vi "read.vi"(8 "error in (no error)":errorcluster caption="错误输入（无错误）", 11 "TCP_client 输入":refnum<class "TCP_client.lvclass">) -> (0 "error out":errorcluster caption="错误输出", 2 "read":string, 3 "TCP_client 输出":refnum<class "TCP_client.lvclass">)   [LabVIEW 2022 SP3, in "update.lvlib" / "TCP_client.lvclass"]
uses:
  TCP_client.lvclass
  TCP_client.lvclass/TCP_client.ctl
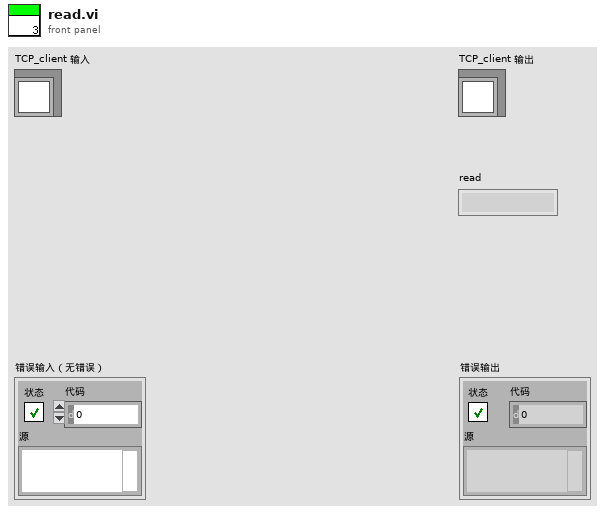
[diagram p1: front panel]
types:
  T1 = enum16{"Standard", "Buffered", "CRLF", "Immediate"}
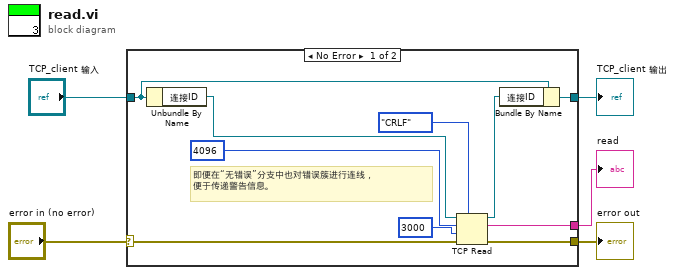
[diagram p0: block diagram]
diagram:
  n1 = case shown="No Error" "error in (no error)" {
    selector: "error in (no error)" -> [w14 w17]
    tunnel: [w13 w17] -> w4
    tunnel: [w9 w16] -> w2
    tunnel: "TCP_client 输入" -> [w11 w16]
    tunnel: [w12 _] -> w1
    frame No Error {
      # "即便在“无错误”分支中也对错误簇进行连线，\n便于传递警告信息。"
      n2 = Unbundle By Name(w11) -> ("连接ID"=w15:refnum<k5>)
      n3 = TCP Read(connection ID=w15, bytes to read=4096 ("读取的字节"), error in (no error)=w14, 7:T1."CRLF" ("模式（标准）"), 9:3000 ("超时毫秒(25000)")) -> (connection ID out=w10:refnum<k5>, data out=w12:string, error out=w13:errorcluster)
      n4 = Bundle By Name(cluster=w11, "连接ID"=w10) -> (w9:refnum<class "TCP_client.lvclass">)
    }
    frame Error {
    }
  }
  "error out" <- w4
  "TCP_client 输出" <- w2
  "read" <- w1
